vi "TSCAN LoadDBC.vi"(0 "路径输入":path, 1 "ADBCAbsolutePath":path=path "C:/Users/DYR/Desktop/M110.dbc", 5 "AIdIn":i32, 9 "ABindChannels":i32[](array[ring])=[0] items=["CHN1", "CHN2", "CHN3", "CHN4", "CHN5", "CHN6", "CHN7", "CHN8", "CHN9", "CHN10", "CHN11", "CHN12", "CHN13", "CHN14", "CHN15", "CHN16", "CHN17", "CHN18", "CHN19", "CHN20", "CHN21", "CHN22", "CHN23", "CHN24", "CHN25", "CHN26", "CHN27", "CHN28", "CHN29", "CHN30", "CHN31", "CHN32"], 11 "错误输入（无错误）":errorcluster) -> (4 "路径输出":path, 6 "AIdOut":i32, 14 "DBC Data":T1 {"ID" format="%x"}, 15 "错误输出":errorcluster)   [LabVIEW 2013]
uses:
  <vilib>/Utility/importsl/GetValueByPointer/datatype.ctl
  <vilib>/Utility/importsl/GetValueByPointer/GetValueByPointer.xnode
panel:
  out "1DSignalName":string[](array[string])
  out "Message&ID":string[](array[string])
  out "ID":i32[](array[numeric]) format="%x"
  out "Message":string[](array[string])
  out "2DSignalName":string[][](array[string])
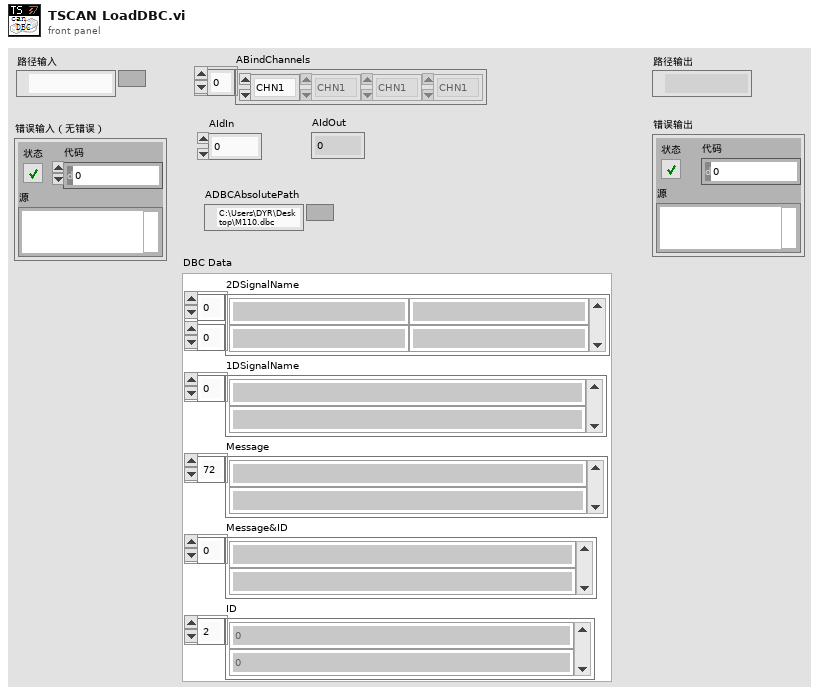
[diagram p1: front panel]
types:
  T1 = cluster{"2DSignalName":string[][], "1DSignalName":string[], "Message":string[], "Message&ID":string[], "ID":i32[]}
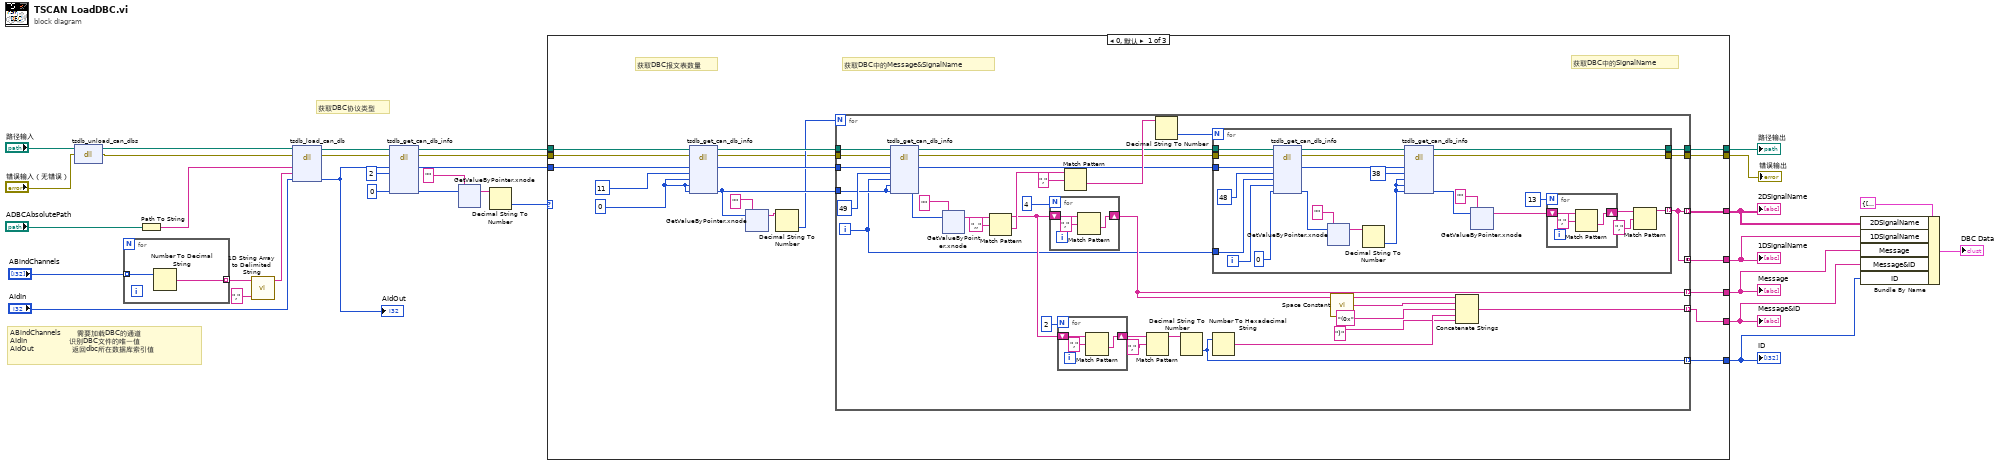
[diagram p0: block diagram]
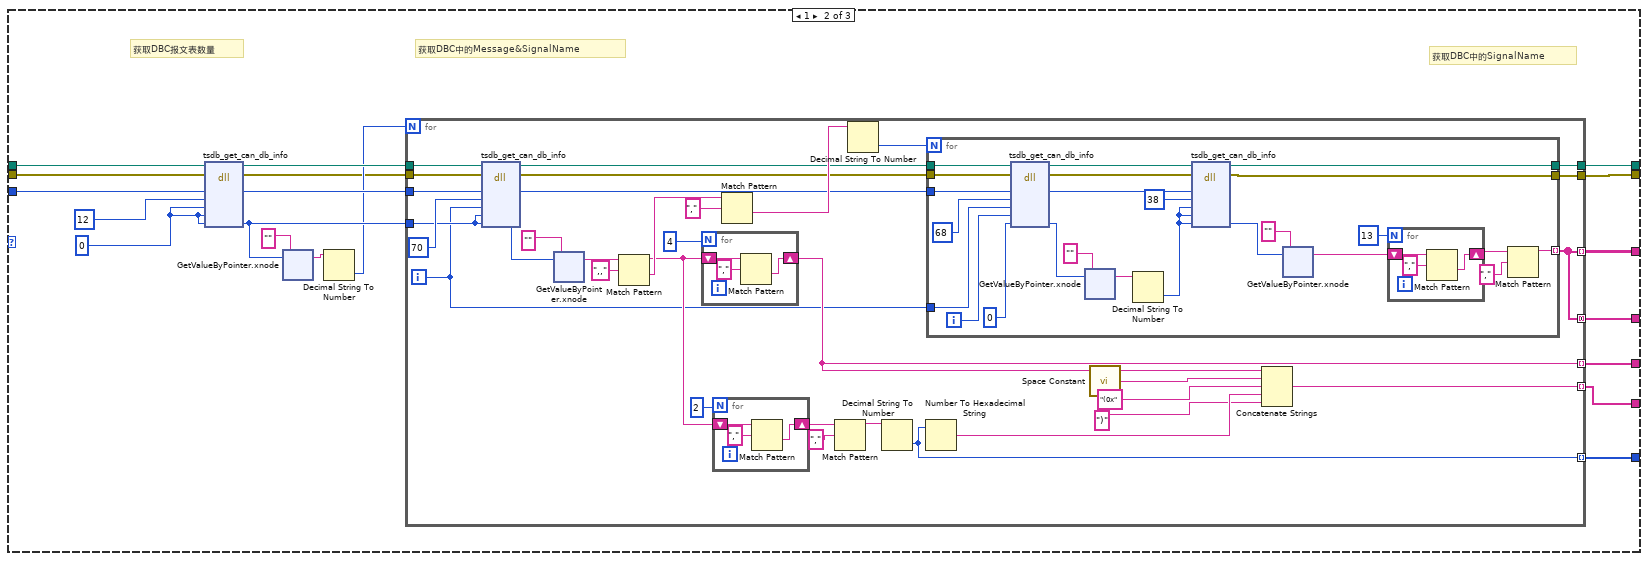
[diagram p2: hidden frame]
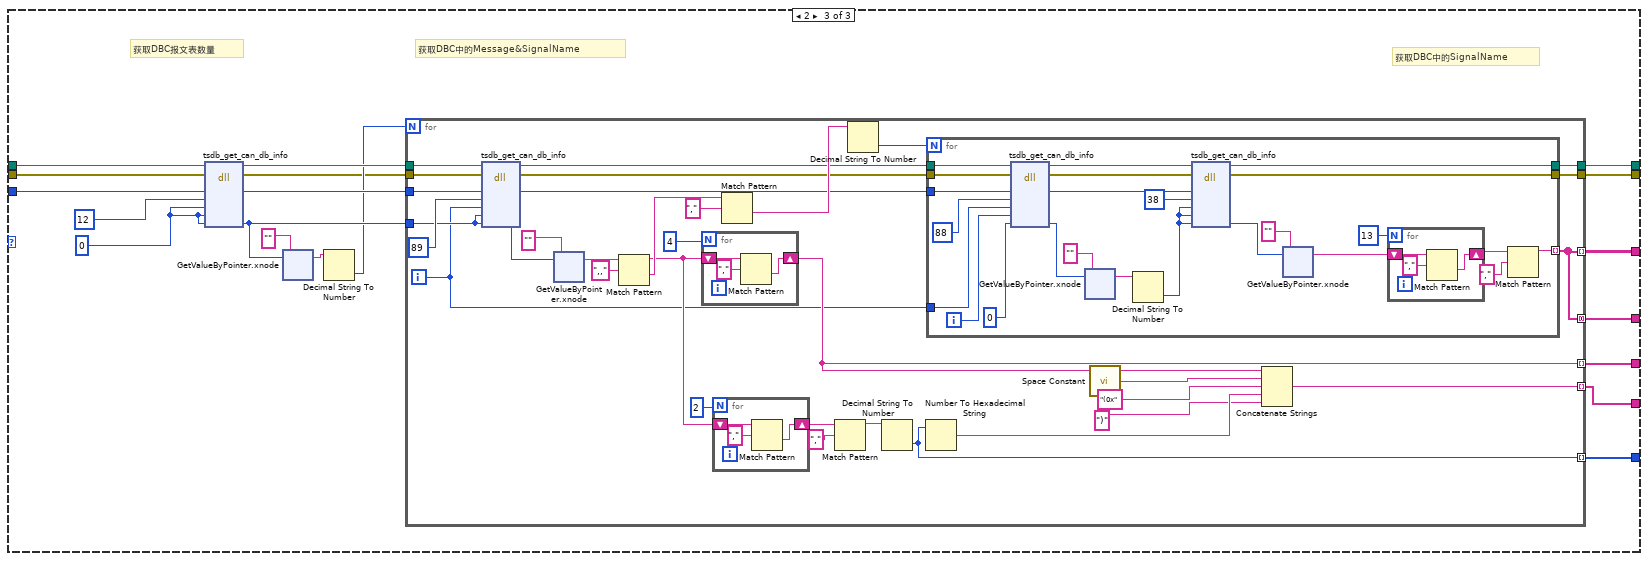
[diagram p3: hidden frame]
diagram:
  w19 = 0 ("AIndex")
  # "获取DBC协议类型"
  # "ABindChannels        需要加载DBC的通道\nAIdIn                     识别DBC文件的唯一值\nAIdOut                   返回dbc所在数据库索引值"
  n1 = dll-call lib="PTH17abs EDemo同星\nTSCAN_V1.0ConfigTSMaster.dll" fn="tsdb_unload_can_dbs"(path in="路径输入", error in="错误输入（无错误）") -> (path out=w24:path, error out=w11:errorcluster)  [unwired: 2 in]
  n2 = for {
    tunnel: "ABindChannels" -> [w34] mode=indexing
    tunnel: [w33] -> w28 mode=indexing
    n3 = Number To Decimal String(number=w34) -> (decimal integer string=w33:string)  [unwired: 1 in]
  }
  n4 = Path To String(path="ADBCAbsolutePath") -> (string=w31:string)
  n5 = call <vilib>:"1D String Array to Delimited String.vi"("delimiter"=",", "string array"=w28) -> ("delimited string"=w26:string)  [unwired: 9 in]
  n6 = dll-call lib="PTH17abs EDemo同星\nTSCAN_V1.0ConfigTSMaster.dll" fn="tsdb_load_can_db"(path in=w24, error in=w11, "ADBCAbsolutePath"=w31, "ABindChannels"=w26, "AId"="AIdIn") -> (path out=w16:path, error out=w10:errorcluster, "AId"=w18:i32)  [unwired: 4 in]
  "AIdOut" <- w18
  n7 = dll-call lib="PTH17abs EDemo同星\nTSCAN_V1.0ConfigTSMaster.dll" fn="tsdb_get_can_db_info"(path in=w16, error in=w10, "ADatabaseld"=w18, "AType"=u32 2, "AIndex"=w19, "ASubIndex"=w19, "Return"=w19) -> (path out=w15:path, error out=w9:errorcluster, "ADatabaseld"=w17:u32, "Return"=w20:i32)  [unwired: 5 in]
  n8 = xnode "GetValueByPointer.xnode"("Pointer"=w20, "InputType"="" ("参数6")) -> ("Output"=w22:string)  [unwired: 2 in, 1 out]
  n9 = Decimal String To Number(string=w22) -> (number=w14:i32)  [unwired: 2 in, 1 out]
  n10 = case shown="0, 默认" w14 {
    tunnel: w15 -> [w45 w178 w311]
    tunnel: w17 -> [w44 w177 w310]
    tunnel: [w43 w175 w308] -> w5
    tunnel: [w42 w173 w306] -> w3
    tunnel: [w41 w172 w305] -> w2
    tunnel: [w40 w174 w307] -> w4
    tunnel: [w39 w176 w309] -> w6
    tunnel: [w38 w171 w304] -> w13
    tunnel: w9 -> [w37 w170 w303]
    tunnel: [w35 w168 w301] -> w8
    frame 0, Default {
      w46 = u32 0 ("AIndex")
      # "获取DBC中的SignalName"
      # "获取DBC中的Message&SignalName"
      # "获取DBC报文表数量"
      n11 = dll-call lib="PTH17abs EDemo同星\nTSCAN_V1.0ConfigTSMaster.dll" fn="tsdb_get_can_db_info"(path in=w45, error in=w37, "ADatabaseld"=w44, "AType"=u32 11, "AIndex"=w46, "ASubIndex"=w46, "Return"=w46) -> (path out=w50:path, error out=w36:errorcluster, "ADatabaseld"=w51:u32, "Return"=w49:i32)  [unwired: 5 in]
      n12 = xnode "GetValueByPointer.xnode"("Pointer"=w49, "InputType"="" ("参数6")) -> ("Output"=w48:string)  [unwired: 2 in, 1 out]
      n13 = Decimal String To Number(string=w48) -> (number=w47:i32)  [unwired: 2 in, 1 out]
      n14 = for {
        N: w47 -> [_]
        tunnel: w51 -> [w84]
        tunnel: w50 -> [w83]
        tunnel: w49 -> [w78]
        tunnel: [w65] -> w40 mode=indexing
        tunnel: [w69] -> w41 mode=indexing
        tunnel: [w67] -> w42 mode=indexing
        tunnel: [w58] -> w39 mode=indexing
        tunnel: [w58] -> w43 mode=concatenating
        tunnel: [w57] -> w38
        tunnel: w36 -> [w56]
        tunnel: [w54] -> w35
        i -> [w60]
        n15 = dll-call lib="PTH17abs EDemo同星\nTSCAN_V1.0ConfigTSMaster.dll" fn="tsdb_get_can_db_info"(path in=w83, error in=w56, "ADatabaseld"=w84, "AType"=u32 49, "AIndex"=w60, "ASubIndex"=w78, "Return"=w78) -> (path out=w61:path, error out=w55:errorcluster, "ADatabaseld"=w59:u32, "Return"=w86:i32)  [unwired: 5 in]
        n16 = xnode "GetValueByPointer.xnode"("Pointer"=w86, "InputType"="" ("参数6")) -> ("Output"=w80:string)  [unwired: 2 in, 1 out]
        n17 = Match Pattern(string=w80, regular expression=",," ("正则表达式")) -> (before substring=w74:string, after substring=w75:string)  [unwired: 1 in, 2 out]
        n18 = for {
          N: 4 -> [_]
          shift-right: [w141] -> w65
          shift-left: w74 -> [w143]
          n19 = Match Pattern(string=w143, regular expression="," ("正则表达式")) -> (after substring=w141:string)  [unwired: 1 in, 3 out]
        }
        n20 = for {
          N: 2 -> [_]
          shift-right: [w138] -> w72
          shift-left: w74 -> [w140]
          n21 = Match Pattern(string=w140, regular expression="," ("正则表达式")) -> (after substring=w138:string)  [unwired: 1 in, 3 out]
        }
        n22 = Match Pattern(string=w75, regular expression="," ("正则表达式")) -> (after substring=w63:string)  [unwired: 1 in, 3 out]
        n23 = Match Pattern(string=w72, regular expression="," ("正则表达式")) -> (before substring=w70:string)  [unwired: 1 in, 3 out]
        n24 = Decimal String To Number(string=w63) -> (number=w62:i32)  [unwired: 2 in, 1 out]
        n25 = Decimal String To Number(string=w70) -> (number=w69:i32)  [unwired: 2 in, 1 out]
        n26 = Number To Hexadecimal String(2:w69) -> (0:w68:string)  [unwired: 1 in]
        n27 = for {
          N: w62 -> [_]
          tunnel: w61 -> [w110]
          tunnel: w59 -> [w109]
          tunnel: [w102] -> w58 mode=indexing
          tunnel: w60 -> [w99]
          tunnel: [w90] -> w57
          tunnel: w55 -> [w89]
          tunnel: [w87] -> w54
          i -> [w100]
          n28 = dll-call lib="PTH17abs EDemo同星\nTSCAN_V1.0ConfigTSMaster.dll" fn="tsdb_get_can_db_info"(path in=w110, error in=w89, "ADatabaseld"=w109, "AType"=u32 48, "AIndex"=w99, "ASubIndex"=w100, "Return"=0 ("ASubIndex")) -> (path out=w97:path, error out=w88:errorcluster, "ADatabaseld"=w96:u32, "Return"=w106:i32)  [unwired: 5 in]
          n29 = xnode "GetValueByPointer.xnode"("Pointer"=w106, "InputType"="" ("参数6")) -> ("Output"=w98:string)  [unwired: 2 in, 1 out]
          n30 = Decimal String To Number(string=w98) -> (number=w94:i32)  [unwired: 2 in, 1 out]
          n31 = dll-call lib="PTH17abs EDemo同星\nTSCAN_V1.0ConfigTSMaster.dll" fn="tsdb_get_can_db_info"(path in=w97, error in=w88, "ADatabaseld"=w96, "AType"=u32 38, "AIndex"=w94, "ASubIndex"=w94, "Return"=w94) -> (path out=w90:path, error out=w87:errorcluster, "Return"=w92:i32)  [unwired: 6 in]
          n32 = xnode "GetValueByPointer.xnode"("Pointer"=w92, "InputType"="" ("参数6")) -> ("Output"=w91:string)  [unwired: 2 in, 1 out]
          n33 = for {
            N: 13 -> [_]
            shift-right: [w123] -> w104
            shift-left: w91 -> [w125]
            n34 = Match Pattern(string=w125, regular expression="," ("正则表达式")) -> (after substring=w123:string)  [unwired: 1 in, 3 out]
          }
          n35 = Match Pattern(string=w104, regular expression="," ("正则表达式")) -> (before substring=w102:string)  [unwired: 1 in, 3 out]
        }
        n36 = call <vilib>:"Space Constant.vi"() -> ("String"=w64:string)
        n37 = Concatenate Strings(w65, w64, "(0x" ("字符串"), w68, ")" ("字符串")) -> (w67:string)
      }
    }
    frame 1 {
      w179 = u32 0 ("AIndex")
      # "获取DBC中的SignalName"
      # "获取DBC中的Message&SignalName"
      # "获取DBC报文表数量"
      n38 = dll-call lib="PTH17abs EDemo同星\nTSCAN_V1.0ConfigTSMaster.dll" fn="tsdb_get_can_db_info"(path in=w178, error in=w170, "ADatabaseld"=w177, "AType"=u32 12, "AIndex"=w179, "ASubIndex"=w179, "Return"=w179) -> (path out=w183:path, error out=w169:errorcluster, "ADatabaseld"=w184:u32, "Return"=w182:i32)  [unwired: 5 in]
      n39 = xnode "GetValueByPointer.xnode"("Pointer"=w182, "InputType"="" ("参数6")) -> ("Output"=w181:string)  [unwired: 2 in, 1 out]
      n40 = Decimal String To Number(string=w181) -> (number=w180:i32)  [unwired: 2 in, 1 out]
      n41 = for {
        N: w180 -> [_]
        tunnel: w184 -> [w217]
        tunnel: w183 -> [w216]
        tunnel: w182 -> [w211]
        tunnel: [w198] -> w174 mode=indexing
        tunnel: [w202] -> w172 mode=indexing
        tunnel: [w200] -> w173 mode=indexing
        tunnel: [w191] -> w176 mode=indexing
        tunnel: [w191] -> w175 mode=concatenating
        tunnel: [w190] -> w171
        tunnel: w169 -> [w189]
        tunnel: [w187] -> w168
        i -> [w193]
        n42 = dll-call lib="PTH17abs EDemo同星\nTSCAN_V1.0ConfigTSMaster.dll" fn="tsdb_get_can_db_info"(path in=w216, error in=w189, "ADatabaseld"=w217, "AType"=u32 70, "AIndex"=w193, "ASubIndex"=w211, "Return"=w211) -> (path out=w194:path, error out=w188:errorcluster, "ADatabaseld"=w192:u32, "Return"=w219:i32)  [unwired: 5 in]
        n43 = xnode "GetValueByPointer.xnode"("Pointer"=w219, "InputType"="" ("参数6")) -> ("Output"=w213:string)  [unwired: 2 in, 1 out]
        n44 = Match Pattern(string=w213, regular expression=",," ("正则表达式")) -> (before substring=w207:string, after substring=w208:string)  [unwired: 1 in, 2 out]
        n45 = for {
          N: 4 -> [_]
          shift-right: [w274] -> w198
          shift-left: w207 -> [w276]
          n46 = Match Pattern(string=w276, regular expression="," ("正则表达式")) -> (after substring=w274:string)  [unwired: 1 in, 3 out]
        }
        n47 = for {
          N: 2 -> [_]
          shift-right: [w271] -> w205
          shift-left: w207 -> [w273]
          n48 = Match Pattern(string=w273, regular expression="," ("正则表达式")) -> (after substring=w271:string)  [unwired: 1 in, 3 out]
        }
        n49 = Match Pattern(string=w208, regular expression="," ("正则表达式")) -> (after substring=w196:string)  [unwired: 1 in, 3 out]
        n50 = Match Pattern(string=w205, regular expression="," ("正则表达式")) -> (before substring=w203:string)  [unwired: 1 in, 3 out]
        n51 = Decimal String To Number(string=w196) -> (number=w195:i32)  [unwired: 2 in, 1 out]
        n52 = Decimal String To Number(string=w203) -> (number=w202:i32)  [unwired: 2 in, 1 out]
        n53 = Number To Hexadecimal String(2:w202) -> (0:w201:string)  [unwired: 1 in]
        n54 = for {
          N: w195 -> [_]
          tunnel: w194 -> [w243]
          tunnel: w192 -> [w242]
          tunnel: [w235] -> w191 mode=indexing
          tunnel: w193 -> [w232]
          tunnel: [w223] -> w190
          tunnel: w188 -> [w222]
          tunnel: [w220] -> w187
          i -> [w233]
          n55 = dll-call lib="PTH17abs EDemo同星\nTSCAN_V1.0ConfigTSMaster.dll" fn="tsdb_get_can_db_info"(path in=w243, error in=w222, "ADatabaseld"=w242, "AType"=u32 68, "AIndex"=w232, "ASubIndex"=w233, "Return"=0 ("ASubIndex")) -> (path out=w230:path, error out=w221:errorcluster, "ADatabaseld"=w229:u32, "Return"=w239:i32)  [unwired: 5 in]
          n56 = xnode "GetValueByPointer.xnode"("Pointer"=w239, "InputType"="" ("参数6")) -> ("Output"=w231:string)  [unwired: 2 in, 1 out]
          n57 = Decimal String To Number(string=w231) -> (number=w227:i32)  [unwired: 2 in, 1 out]
          n58 = dll-call lib="PTH17abs EDemo同星\nTSCAN_V1.0ConfigTSMaster.dll" fn="tsdb_get_can_db_info"(path in=w230, error in=w221, "ADatabaseld"=w229, "AType"=u32 38, "AIndex"=w227, "ASubIndex"=w227, "Return"=w227) -> (path out=w223:path, error out=w220:errorcluster, "Return"=w225:i32)  [unwired: 6 in]
          n59 = xnode "GetValueByPointer.xnode"("Pointer"=w225, "InputType"="" ("参数6")) -> ("Output"=w224:string)  [unwired: 2 in, 1 out]
          n60 = for {
            N: 13 -> [_]
            shift-right: [w256] -> w237
            shift-left: w224 -> [w258]
            n61 = Match Pattern(string=w258, regular expression="," ("正则表达式")) -> (after substring=w256:string)  [unwired: 1 in, 3 out]
          }
          n62 = Match Pattern(string=w237, regular expression="," ("正则表达式")) -> (before substring=w235:string)  [unwired: 1 in, 3 out]
        }
        n63 = call <vilib>:"Space Constant.vi"() -> ("String"=w197:string)
        n64 = Concatenate Strings(w198, w197, "(0x" ("字符串"), w201, ")" ("字符串")) -> (w200:string)
      }
    }
    frame 2 {
      w312 = u32 0 ("AIndex")
      # "获取DBC中的SignalName"
      # "获取DBC中的Message&SignalName"
      # "获取DBC报文表数量"
      n65 = dll-call lib="PTH17abs EDemo同星\nTSCAN_V1.0ConfigTSMaster.dll" fn="tsdb_get_can_db_info"(path in=w311, error in=w303, "ADatabaseld"=w310, "AType"=u32 12, "AIndex"=w312, "ASubIndex"=w312, "Return"=w312) -> (path out=w316:path, error out=w302:errorcluster, "ADatabaseld"=w317:u32, "Return"=w315:i32)  [unwired: 5 in]
      n66 = xnode "GetValueByPointer.xnode"("Pointer"=w315, "InputType"="" ("参数6")) -> ("Output"=w314:string)  [unwired: 2 in, 1 out]
      n67 = Decimal String To Number(string=w314) -> (number=w313:i32)  [unwired: 2 in, 1 out]
      n68 = for {
        N: w313 -> [_]
        tunnel: w317 -> [w350]
        tunnel: w316 -> [w349]
        tunnel: w315 -> [w344]
        tunnel: [w331] -> w307 mode=indexing
        tunnel: [w335] -> w305 mode=indexing
        tunnel: [w333] -> w306 mode=indexing
        tunnel: [w324] -> w309 mode=indexing
        tunnel: [w324] -> w308 mode=concatenating
        tunnel: [w323] -> w304
        tunnel: w302 -> [w322]
        tunnel: [w320] -> w301
        i -> [w326]
        n69 = dll-call lib="PTH17abs EDemo同星\nTSCAN_V1.0ConfigTSMaster.dll" fn="tsdb_get_can_db_info"(path in=w349, error in=w322, "ADatabaseld"=w350, "AType"=u32 89, "AIndex"=w326, "ASubIndex"=w344, "Return"=w344) -> (path out=w327:path, error out=w321:errorcluster, "ADatabaseld"=w325:u32, "Return"=w352:i32)  [unwired: 5 in]
        n70 = xnode "GetValueByPointer.xnode"("Pointer"=w352, "InputType"="" ("参数6")) -> ("Output"=w346:string)  [unwired: 2 in, 1 out]
        n71 = Match Pattern(string=w346, regular expression=",," ("正则表达式")) -> (before substring=w340:string, after substring=w341:string)  [unwired: 1 in, 2 out]
        n72 = for {
          N: 4 -> [_]
          shift-right: [w407] -> w331
          shift-left: w340 -> [w409]
          n73 = Match Pattern(string=w409, regular expression="," ("正则表达式")) -> (after substring=w407:string)  [unwired: 1 in, 3 out]
        }
        n74 = for {
          N: 2 -> [_]
          shift-right: [w404] -> w338
          shift-left: w340 -> [w406]
          n75 = Match Pattern(string=w406, regular expression="," ("正则表达式")) -> (after substring=w404:string)  [unwired: 1 in, 3 out]
        }
        n76 = Match Pattern(string=w341, regular expression="," ("正则表达式")) -> (after substring=w329:string)  [unwired: 1 in, 3 out]
        n77 = Match Pattern(string=w338, regular expression="," ("正则表达式")) -> (before substring=w336:string)  [unwired: 1 in, 3 out]
        n78 = Decimal String To Number(string=w329) -> (number=w328:i32)  [unwired: 2 in, 1 out]
        n79 = Decimal String To Number(string=w336) -> (number=w335:i32)  [unwired: 2 in, 1 out]
        n80 = Number To Hexadecimal String(2:w335) -> (0:w334:string)  [unwired: 1 in]
        n81 = for {
          N: w328 -> [_]
          tunnel: w327 -> [w376]
          tunnel: w325 -> [w375]
          tunnel: [w368] -> w324 mode=indexing
          tunnel: w326 -> [w365]
          tunnel: [w356] -> w323
          tunnel: w321 -> [w355]
          tunnel: [w353] -> w320
          i -> [w366]
          n82 = dll-call lib="PTH17abs EDemo同星\nTSCAN_V1.0ConfigTSMaster.dll" fn="tsdb_get_can_db_info"(path in=w376, error in=w355, "ADatabaseld"=w375, "AType"=u32 88, "AIndex"=w365, "ASubIndex"=w366, "Return"=0 ("ASubIndex")) -> (path out=w363:path, error out=w354:errorcluster, "ADatabaseld"=w362:u32, "Return"=w372:i32)  [unwired: 5 in]
          n83 = xnode "GetValueByPointer.xnode"("Pointer"=w372, "InputType"="" ("参数6")) -> ("Output"=w364:string)  [unwired: 2 in, 1 out]
          n84 = Decimal String To Number(string=w364) -> (number=w360:i32)  [unwired: 2 in, 1 out]
          n85 = dll-call lib="PTH17abs EDemo同星\nTSCAN_V1.0ConfigTSMaster.dll" fn="tsdb_get_can_db_info"(path in=w363, error in=w354, "ADatabaseld"=w362, "AType"=u32 38, "AIndex"=w360, "ASubIndex"=w360, "Return"=w360) -> (path out=w356:path, error out=w353:errorcluster, "Return"=w358:i32)  [unwired: 6 in]
          n86 = xnode "GetValueByPointer.xnode"("Pointer"=w358, "InputType"="" ("参数6")) -> ("Output"=w357:string)  [unwired: 2 in, 1 out]
          n87 = for {
            N: 13 -> [_]
            shift-right: [w389] -> w370
            shift-left: w357 -> [w391]
            n88 = Match Pattern(string=w391, regular expression="," ("正则表达式")) -> (after substring=w389:string)  [unwired: 1 in, 3 out]
          }
          n89 = Match Pattern(string=w370, regular expression="," ("正则表达式")) -> (before substring=w368:string)  [unwired: 1 in, 3 out]
        }
        n90 = call <vilib>:"Space Constant.vi"() -> ("String"=w330:string)
        n91 = Concatenate Strings(w331, w330, "(0x" ("字符串"), w334, ")" ("字符串")) -> (w333:string)
      }
    }
  }
  "2DSignalName" <- w6
  "Message" <- w4
  "ID" <- w2
  "Message&ID" <- w3
  "1DSignalName" <- w5
  "路径输出" <- w13
  "错误输出" <- w8
  n92 = Bundle By Name(cluster=T1 {"2DSignalName"=[], "1DSignalName"=[], "Message"=[], "Message&ID"=[], "ID"=[]} ("DBC Data"), "2DSignalName"=w6, "1DSignalName"=w5, "Message"=w4, "Message&ID"=w3, "ID"=w2) -> (→"DBC Data":T1)
